vi "Test Launcher AF Configurable.vi"   [LabVIEW 2014]
uses:
  ConfigurableActor/ConfigurableActor.lvclass/ConfigurableActor.ctl
  <vilib>/ActorFramework/Message Enqueuer/Message Enqueuer.lvclass/Message Enqueuer.ctl
  <vilib>/ActorFramework/Message Enqueuer/Enqueue.vi
  <vilib>/ActorFramework/Message Priority Queue/Priority Enqueue.vi
  <vilib>/ActorFramework/Stop Msg/Stop Msg.lvclass
  <vilib>/ActorFramework/Actor/Actor.lvclass
  ConfigurableActor/ConfigurableActor.lvclass
panel:
  # "System Level UI"
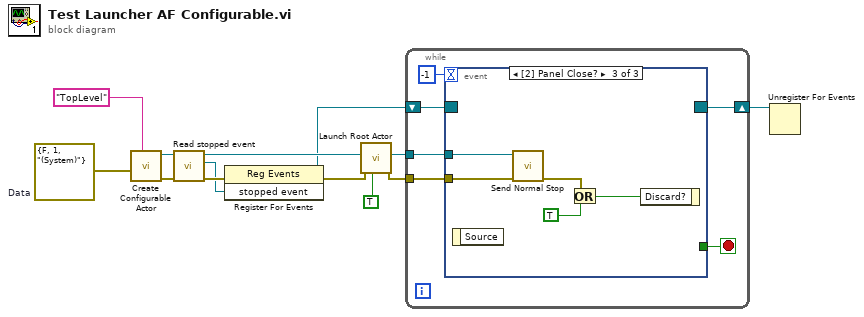
[diagram p0: block diagram]
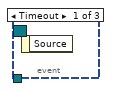
[diagram p2: hidden frame]
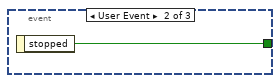
[diagram p3: hidden frame]
diagram:
  w1 = errorcluster {"status"=FALSE, "code"=1, "source"="(System)"}  # Data
  n1 = call "Create Configurable Actor.vi"("Name"="TopLevel", "Configuration"=w1) -> ("error out"=w9:errorcluster, "ConfigurableActor out"=w11:refnum<class "ConfigurableActor.lvclass">)  [unwired: 8 in]
  n2 = call "Read stopped event.vi"("error in (no error)"=w9, "ConfigurableActor in"=w11) -> ("error out"=w8:errorcluster, "stopped event"=w7:refnum<user-event>, "ConfigurableActor out"=w10:refnum<class "ConfigurableActor.lvclass">)  [unwired: 7 in]
  n3 = register-events(error in=w8, w7) -> (reference out=w4:refnum<event-registration>, error out=w6:errorcluster)  [unwired: 1 in]
  n4 = call <vilib>:"Launch Root Actor.vi"("Open Actor Core front panel? (F)"=TRUE, "error in (no error)"=w6, "Actor"=w10) -> ("error out"=w5:errorcluster, "Actor's Enqueuer"=w13:refnum<class "Message Enqueuer.lvclass">)  [unwired: 7 in]
  n5 = while {
    tunnel: w13 -> [w18]
    tunnel: w5 -> [w16]
    shift-right: [w14] -> w3
    shift-left: w4 -> [w15]
    stop <- w17 stop-if-true
    n6 = event shown="[2] Panel Close?" {
      selector: w15 -> [_ _ _]
      dyn-events: [_ _ _] -> w14
      timeout: -1 -> [_ _ _]
      tunnel: w18 -> [_ _ w25]
      tunnel: [_ w20 _] -> w17
      tunnel: w16 -> [_ _ w21]
      event Timeout {
        n7 = event-data() -> ()  [unwired: 1 in, 1 out]
      }
      event User Event {
        n8 = event-data() -> ("stopped"=w20:bool)  [unwired: 1 in]
      }
      event Panel Close? {
        n9 = event-data() -> ()  [unwired: 1 in, 1 out]
        n10 = call <vilib>:"Send Normal Stop.vi"("error in (no error)"=w21, "Message Enqueuer"=w25) -> ("error out"=w24:errorcluster)  [unwired: 9 in]
        n11 = Or(x=w24, y=TRUE ("Discard?")) -> (x .or. y?=w22:bool)
        n12 = event-data("Discard?"=w22) -> ()  [unwired: 1 in, 1 out]
      }
    }
  }
  n13 = Unregister For Events(event registration refnum=w3) -> ()  [unwired: 1 in, 1 out]
